vi "Photometric values.vi"(8 "error in (no error)":errorcluster, 10 "Power Spectral Distribution":cluster{"X":dbl, "Y":dbl}[](graph), 11 "Hardware Resources in":T1) -> (0 "error out":errorcluster, 2 "Color Parameters out":T5 {"Color Values"."v'" format="%#_5g"; "Color Values"."Duv" format="%#_5g"; "Color Values"."u'" format="%#_5g"; "Color Values"."CRI" format="%#_5g"; "Color Values"."CCT" format="%#_5g"; "Color Values"."luminousFlux" format="%#_5g"; "R values" format="%#_4g"; "Tristimulus \nValues"."Z" format="%#_5g"; "Tristimulus \nValues"."Y" format="%#_5g"; "Tristimulus \nValues"."X" format="%#_5g"; "Chromaticity \nCoordinates"."v" format="%#_5g"; "Chromaticity \nCoordinates"."u" format="%#_5g"; "Chromaticity \nCoordinates"."z" format="%#_5g"; "Chromaticity \nCoordinates"."y" format="%#_5g"; "Chromaticity \nCoordinates"."x" format="%#_5g"})   [LabVIEW 2014, in "AvaSpec.lvlib"]
doc: "Determines the different color parameters (lumens, CCT, CRI, duv, etc.) based on the input spectrum"
uses:
  AvaSpec.lvlib
  Acquisition/AvaSpec Color Parameters.ctl
  Acquisition/Sphere Indicator.ctl
  Acquisition/Hardware Configuration.ctl
  AS-5216-DLL/AVS settings.ctl
  Settings/Measurement Type.ctl
  IRRAD input parameters.ctl
  AVSirrad_support.lvlib
  Acquisition/AvaSpec Acquisition.lvlib
panel:
  # "Input"
  # "Output"
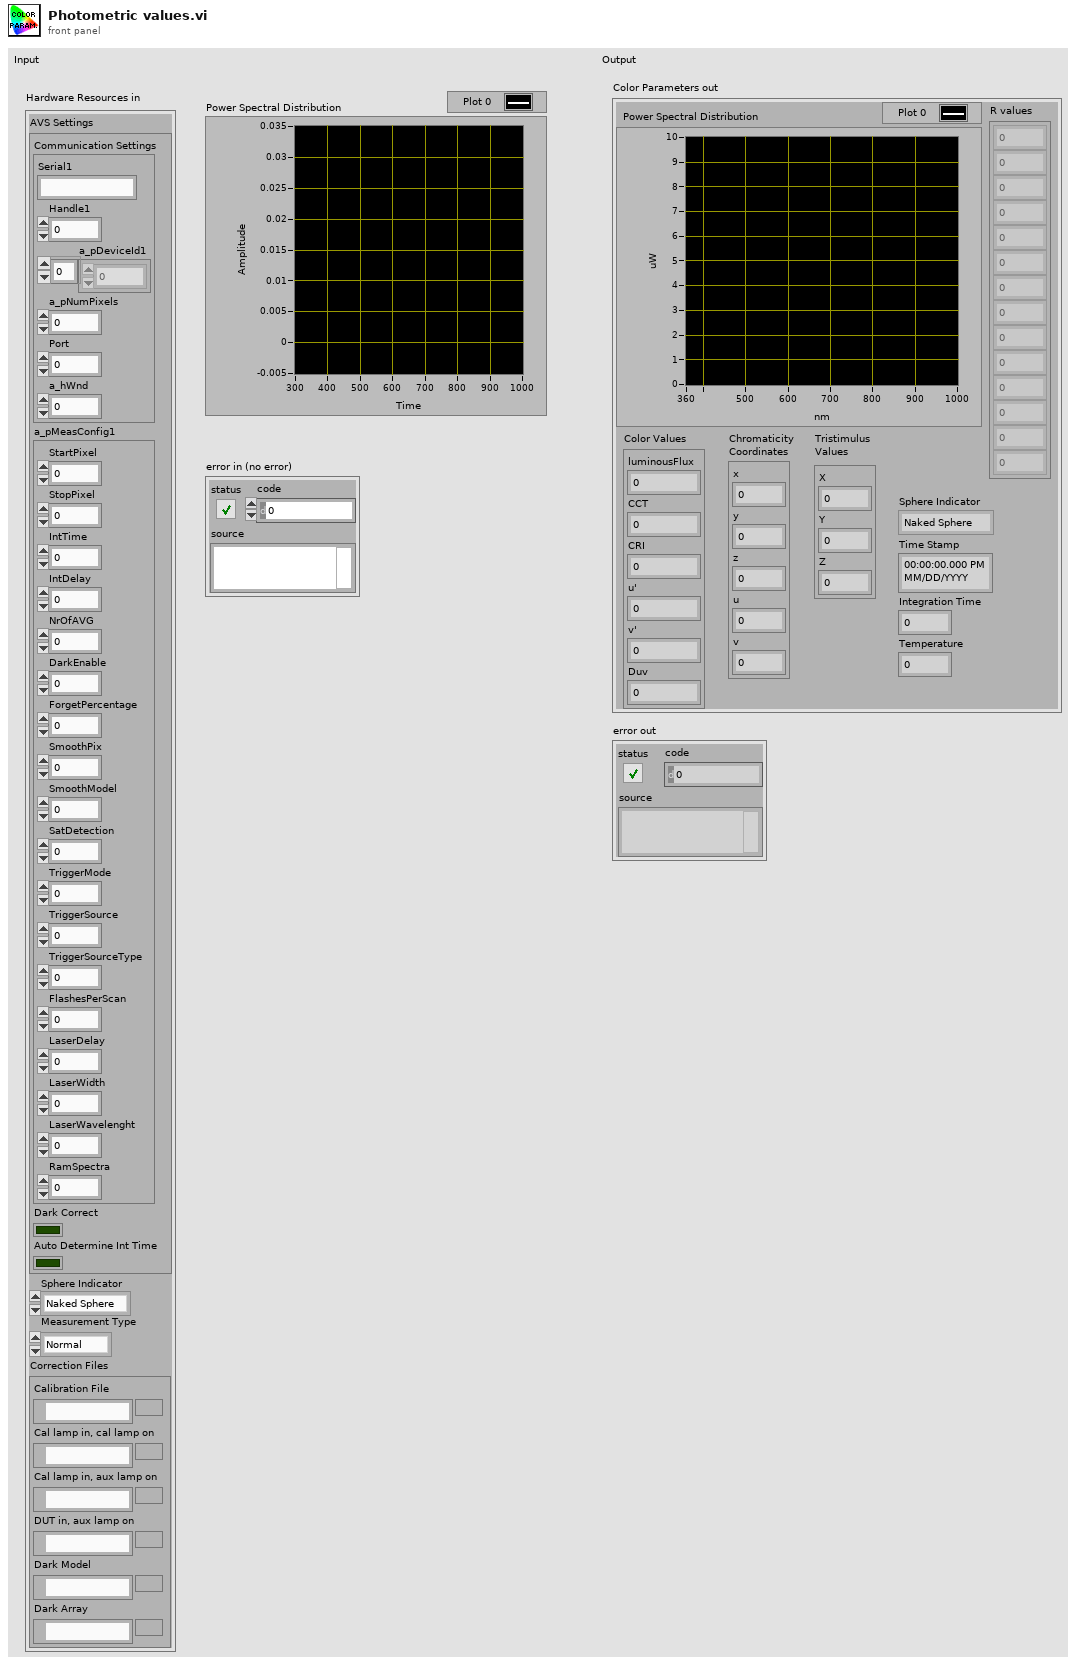
[diagram p1: front panel]
types:
  T1 = typedef "AvaSpec.lvlib/AvaSpec Acquisition.lvlib/Hardware Configuration.ctl" = cluster{"AVS Settings":T2, "Sphere Indicator":T3, "Measurement Type":T4, "Correction Files":cluster{"Calibration File":path, "Cal lamp in, cal lamp on":path, "Cal lamp in, aux lamp on":path, "DUT in, aux lamp on":path, "Dark Model":path, "Dark Array":path}}
  T2 = typedef "AvaSpec.lvlib/AVS settings.ctl" = cluster{"Communication Settings":cluster{"Serial1":string, "Handle1":i32, "a_pDeviceId1":u8[], "a_pNumPixels":u16, "Port":i32, "a_hWnd":i32}, "a_pMeasConfig1":cluster{"StartPixel":u16, "StopPixel":u16, "IntTime":sgl, "IntDelay":u32, "NrOfAVG":u32, "DarkEnable":u8, "ForgetPercentage":u8, "SmoothPix":u16, "SmoothModel":u8, "SatDetection":u8, "TriggerMode":u8, "TriggerSource":u8, "TriggerSourceType":u8, "FlashesPerScan":u16, "LaserDelay":u32, "LaserWidth":u32, "LaserWavelenght":sgl, "RamSpectra":u16}, "Dark Correct":bool, "Auto Determine Int Time":bool}
  T3 = typedef "AvaSpec.lvlib/Sphere Indicator.ctl" = enum16{"Naked Sphere", "Insulated Sphere"}
  T4 = typedef "AvaSpec.lvlib/AvaSpec Acquisition.lvlib/Measurement Type.ctl" = enum16{"Normal", "Calibration", "Dark"}
  T5 = typedef "AvaSpec.lvlib/AvaSpec Color Parameters.ctl" = cluster{"Power Spectral Distribution":cluster{"X":dbl, "Y":dbl}[], "Color Values":cluster{"luminousFlux":dbl, "CCT":dbl, "CRI":dbl, "u'":dbl, "v'":dbl, "Duv":dbl}, "R values":dbl[], "Chromaticity \nCoordinates":cluster{"x":dbl, "y":dbl, "z":dbl, "u":dbl, "v":dbl}, "Tristimulus \nValues":cluster{"X":dbl, "Y":dbl, "Z":dbl}, "Time Stamp":timestamp, "Temperature":dbl, "Integration Time":dbl, "Sphere Indicator":T3}
  T6 = typedef "AvaSpec.lvlib/IRRAD input parameters.ctl" = cluster{"a_data":dbl[], "num_points":i32, "a_Observer":u8, "a_CIEResolution":u8}
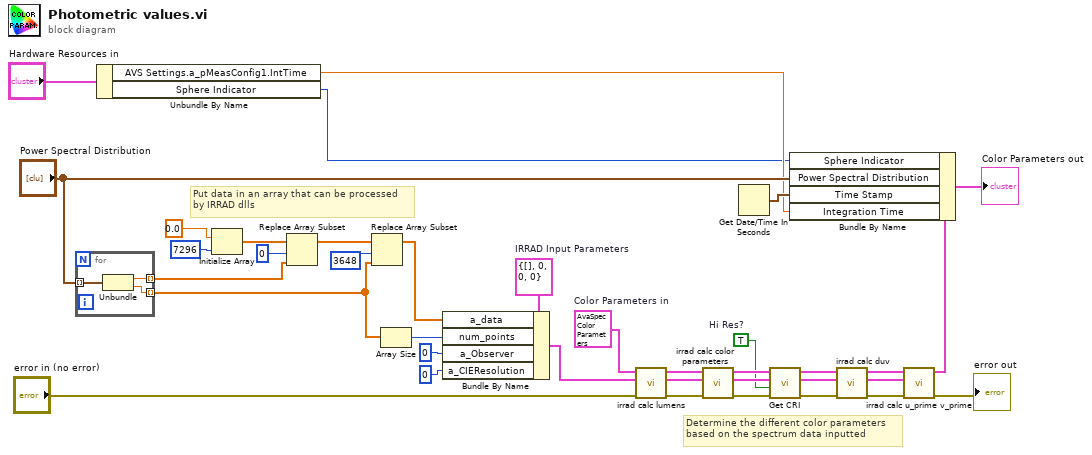
[diagram p0: block diagram]
diagram:
  w22 = T6 {"a_data"=[], "num_points"=0, "a_Observer"=0, "a_CIEResolution"=0}  # IRRAD Input Parameters
  w17 = TRUE  # Hi Res?
  w20 = T5 {"Power Spectral Distribution"=[], "Color Values"={"luminousFlux"=0.0, "CCT"=0.0, "CRI"=0.0, "u'"=0.0, "v'"=0.0, "Duv"=0.0}, "R values"=[], "Chromaticity \nCoordinates"={"x"=0.0, "y"=0.0, "z"=0.0, "u"=0.0, "v"=0.0}, "Tristimulus \nValues"={"X"=0.0, "Y"=0.0, "Z"=0.0}, "Time Stamp"=timestamp(0 s since 1904-01-01), "Temperature"=0.0, "Integration Time"=0.0, "Sphere Indicator"=enum."Naked Sphere"}  # Color Parameters in
  # "Determine the different color parameters\nbased on the spectrum data inputted"
  # "Put data in an array that can be processed\nby IRRAD dlls"
  n1 = for {
    tunnel: "Power Spectral Distribution" -> [w40] mode=indexing
    tunnel: [w39] -> w32 mode=indexing
    tunnel: [w38] -> w33 mode=indexing
    n2 = Unbundle(w40) -> ("X"=w38:dbl, "Y"=w39:dbl)
  }
  n3 = Unbundle By Name("Hardware Resources in") -> ("AVS Settings.a_pMeasConfig1.IntTime"=w2:sgl, "Sphere Indicator"=w1:T3)
  n4 = Initialize Array(0.0 ("element"), 7296 ("dimension size")) -> (w36:dbl[])
  n5 = Replace Array Subset(array=w36, new element=w33, index=0) -> (w37:dbl[])
  n6 = Replace Array Subset(array=w37, new element=w32, index=3648 ("dimension size")) -> (w19:dbl[])
  n7 = Array Size(array=w32) -> (size(s)=w18:i32)
  n8 = Bundle By Name(cluster=w22, "a_data"=w19, "num_points"=w18, "a_Observer"=u8 0, "a_CIEResolution"=u8 0) -> (w21:T6)
  n9 = call "irrad calc lumens.vi"("error in (no error)"="error in (no error)", "IRRAD Input Parameters"=w21, "Color Parameters in"=w20) -> ("error out"=w29:errorcluster, "IRRAD Input Parameters out"=w24:T6, "Color Parameters out"=w27:T5)  [unwired: 6 in]
  n10 = call "irrad calc color parameters.vi"("error in (no error)"=w29, "IRRAD Input Parameters"=w24, "Color Parameters in"=w27) -> ("error out"=w28:errorcluster, "IRRAD Input Parameters out"=w25:T6, "Color Parameters out"=w26:T5)  [unwired: 6 in]
  n11 = Get Date/Time In Seconds() -> (seconds since 1Jan1904=w12:timestamp)
  n12 = call "Get CRI.vi"("error in (no error)"=w28, "Hi Res?"=w17, "IRRAD Input Parameters"=w25, "Color Parameters in"=w26) -> ("error out"=w10:errorcluster, "IRRAD Input Parameters out"=w4:T6, "Color Parameters out"=w11:T5)  [unwired: 5 in]
  n13 = call "irrad calc duv.vi"("error in (no error)"=w10, "IRRAD Input Parameters"=w4, "Color Parameters in"=w11) -> ("error out"=w6:errorcluster, "IRRAD Input Parameters out"=w8:T6, "Color Parameters out"=w9:T5)  [unwired: 6 in]
  n14 = call "irrad calc u_prime v_prime.vi"("error in (no error)"=w6, "IRRAD Input Parameters"=w8, "Color Parameters in"=w9) -> ("error out"=→"error out":errorcluster, "Color Parameters out"=w7:T5)  [unwired: 6 in, 1 out]
  n15 = Bundle By Name(cluster=w7, "Sphere Indicator"=w1, "Power Spectral Distribution"="Power Spectral Distribution", "Time Stamp"=w12, "Integration Time"=w2) -> (→"Color Parameters out":T5)
